vi "ParseXLG.vi"(8 "error in (no error)":errorcluster, 10 "Path":path=path "C:/Users/zong/OneDrive - NI/Desktop/XNET/XCP_otherID/XCP_OtherDTOID/ECUMCLog/XCP or CCP Master_Protocol_Log.txt", 11 "DAQList in":refnum<class "DAQList.lvclass">) -> (0 "error out":errorcluster, 2 "CAN Frames":T1[](array[typedef]) {"payload" format="%x"; "timestamp" format="%<%.7X\n%x>T"; "type" items=["CAN Data"=0, "CAN Remote"=1, "CAN Bus Error"=2, "CAN 2.0 Data"=8, "CAN FD Data"=16, "CAN FD+BRS Data"=24, "J1939 Data"=192, "Delay"=224, "Log Trigger"=225, "Start Trigger"=226]; "identifier" format="%x"}, 3 "DAQList out":refnum<class "DAQList.lvclass">)   [LabVIEW 2019, in "XCP_DaqDtoId.lvlib" / "DAQList.lvclass"]
uses:
  DAQList.lvclass
  <vilib>/xnet/xnet.llb/XNET Frame CAN.ctl
  <vilib>/xnet/xnet.llb/XNET Frame Type CAN.ctl
  DAQList.lvclass/DAQList.ctl
  <vilib>/Utility/file.llb/Read Delimited Spreadsheet (string).vi
  <vilib>/ECUMC/ECUMC.llb/MC Get Prop XCP DTO Id.vi
  <vilib>/ECUMC/ECUMC.llb/MC Get Prop XCP CRO Id.vi
  <vilib>/ECUMC/ECUMC.lvlib
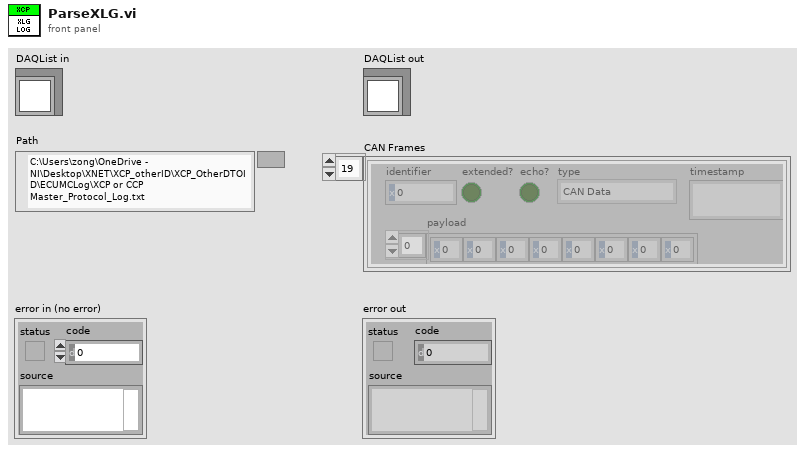
[diagram p1: front panel]
types:
  T1 = typedef "XNET Frame CAN.ctl" = cluster{"timestamp":timestamp, "payload":u8[], "identifier":u32, "type":T2, "extended?":bool, "echo?":bool}
  T2 = typedef "XNET Frame Type CAN.ctl" = u8
  T3 = typedef "ECUMC.lvlib/MC Reference.ctt" = u32
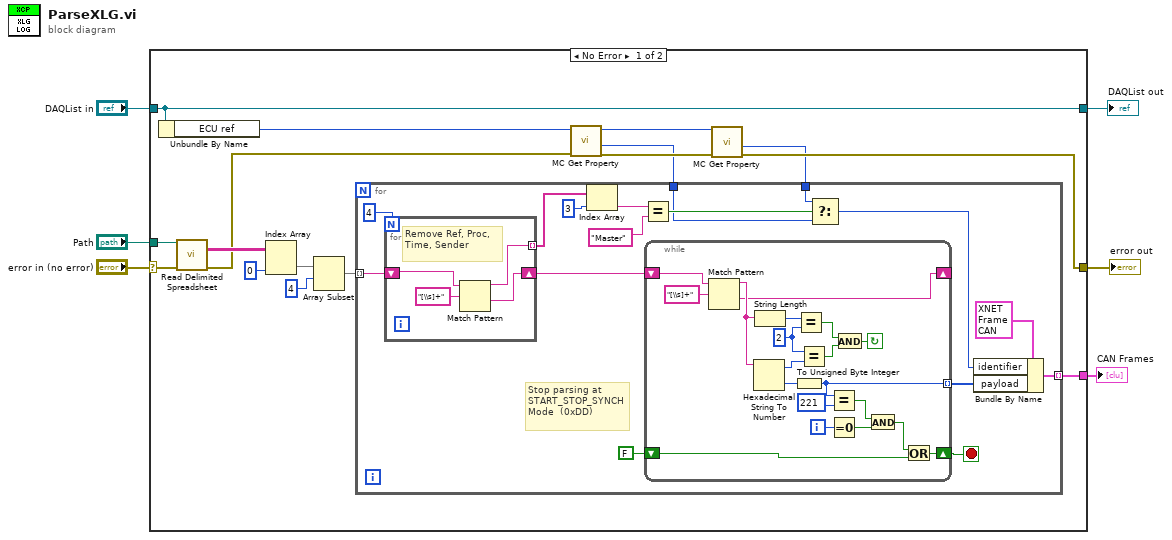
[diagram p0: block diagram]
diagram:
  n1 = case shown="No Error" "error in (no error)" {
    selector: "error in (no error)" -> [w21 w63]
    tunnel: [w9 w63] -> w5
    tunnel: [w14 w62] -> w3
    tunnel: "DAQList in" -> [w14 w62]
    tunnel: "Path" -> [w22 _]
    tunnel: [w15 _] -> w1
    frame No Error {
      n2 = Unbundle By Name(w14) -> ("ECU ref"=w13:T3)
      n3 = call-poly <vilib>:"Read Delimited Spreadsheet.vi"("file path (dialog if empty)"=w22, "error in (no error)"=w21) -> ("all rows"=w19:string[][], "error out"=w10:errorcluster)  [unwired: 8 in, 4 out]
      n4 = Index Array(array=w19, index (col)=0 ("disabled index (col)")) -> (element=w17:string[])  [unwired: 1 in]
      n5 = Array Subset(array=w17, index=4) -> (w16:string[])  [unwired: 1 in]
      n6 = call-poly <vilib>:"MC Get Property.vi"("error in"=w10, "reference in"=w13) -> ("error out"=w11:errorcluster, "XCP DTO id"=w7:u32, "reference out"=w12:T3)  [unwired: 7 in]
      n7 = call-poly <vilib>:"MC Get Property.vi"("error in"=w11, "reference in"=w12) -> ("error out"=w9:errorcluster, "XCP CRO id"=w8:u32)  [unwired: 7 in, 1 out]
      n8 = for {
        tunnel: w16 -> [w36] mode=indexing
        tunnel: [w35] -> w15 mode=indexing
        tunnel: w8 -> [w25]
        tunnel: w7 -> [w24]
        stop <- w34 stop-if-true
        # "Stop parsing at START_STOP_SYNCH Mode  (0xDD)"
        n9 = for {
          N: 4 -> [_]
          shift-right: [w59] -> w37
          shift-left: w36 -> [w61]
          tunnel: [w58] -> w30 mode=indexing
          # "Remove Ref, Proc, Time, Sender"
          n10 = Match Pattern(string=w61, regular expression="[\\s]+") -> (before substring=w58:string, after substring=w59:string)  [unwired: 1 in, 2 out]
        }
        n11 = Index Array(array=w30, index=3) -> (element=w28:string)
        n12 = Equal?(x=w28, y="Master") -> (x = y?=w26:bool)
        n13 = while {
          shift-right: [w48] -> _
          shift-left: w37 -> [w57]
          tunnel: [w45] -> w32 mode=indexing
          shift-right: [w40] -> w34
          shift-left: FALSE -> [w39]
          i -> [w46]
          stop <- w49 continue-if-true
          w53 = 2 ("y")
          n14 = Match Pattern(string=w57, regular expression="[\\s]+") -> (before substring=w54:string, after substring=w48:string)  [unwired: 1 in, 2 out]
          n15 = Hexadecimal String To Number(string=w54) -> (offset past number=w52:i32, number=w47:u32)  [unwired: 2 in]
          n16 = String Length(string=w54) -> (length=w55:i32)
          n17 = To Unsigned Byte Integer(number=w47) -> (unsigned 8bit integer=w45:u8)
          n18 = Equal?(x=w55, y=w53) -> (x = y?=w51:bool)
          n19 = Equal?(x=w53, y=w52) -> (x = y?=w50:bool)
          n20 = Equal?(x=w45, y=u8 221 ("unsigned 8bit integer")) -> (x = y?=w43:bool)
          n21 = Equal To 0?(x=w46) -> (x = 0?=w42:bool)
          n22 = And(x=w51, y=w50) -> (x .and. y?=w49:bool)
          n23 = And(x=w43, y=w42) -> (x .and. y?=w41:bool)
          n24 = Or(x=w41, y=w39) -> (x .or. y?=w40:bool)
        }
        n25 = Select(t=w25, s=w26, f=w24) -> (s? t:f=w23:u32)
        n26 = Bundle By Name(cluster=T1 {"timestamp"=timestamp(0 s since 1904-01-01), "payload"=[], "identifier"=0, "type"=0, "extended?"=FALSE, "echo?"=FALSE} ("CAN frame"), "identifier"=w23, "payload"=w32) -> (w35:T1)
      }
    }
    frame Error {
    }
  }
  "error out" <- w5
  "DAQList out" <- w3
  "CAN Frames" <- w1
